vi "CreateIntegerArray.vi"(1 "Spacing":u16(ring) items=["Linear", "Logorithmic"], 2 "Pts":dbl, 3 "Max":dbl, 4 "Min":dbl) -> (0 "OutputArray":dbl[](array[numeric]))   [LabVIEW 2015]
uses:
  <vilib>/imath/engines/lvmath2/RunTimeSupport/NIMS_Complex To Real.vi
  <instcachedir>/0/NIMS_Complex To Real_01315F44AA8B4CE79FEF95AE999DC25E.lvgen/NIMS_Complex To Real_01315F44AA8B4CE79FEF95AE999DC25E_001.vi
  <vilib>/imath/engines/lvmath2/RunTimeEngine/BuiltInFunctions/logramp/NIMS_logramp.vi
  <vilib>/imath/engines/lvmath2/RunTimeEngine/ErrorHandling/NIMS_Create Error From Enums.vi
  <vilib>/imath/engines/lvmath2/RunTimeEngine/BuiltInFunctions/linramp/NIMS_linramp.vi
  <vilib>/imath/engines/lvmath2/RunTimeEngine/VariableToken/NIMS_VariableToken_CondDefined.vi
  <instcachedir>/0/NIMS_VariableToken_CondDefined_FE30D0A1BFB24F098D41DEBABFE96BE1.lvgen/NIMS_VariableToken_CondDefined_FE30D0A1BFB24F098D41DEBABFE96BE1_003.vi
  <vilib>/imathl/engines/lvmath/Functions/Error Handling/Create Error.vi
  <vilib>/imath/engines/lvmath2/RunTimeEngine/NodeEndStatement/NIMS_NodeEndStatement_Output.vi
  <instcachedir>/0/NIMS_NodeEndStatement_Output_53EC0D466D134D7ABD903AC30B43404B.lvgen/NIMS_NodeEndStatement_Output_53EC0D466D134D7ABD903AC30B43404B_005.vi
  <vilib>/imath/engines/lvmath2/RunTimeEngine/ErrorHandling/NIMS_Finalize Error.vi
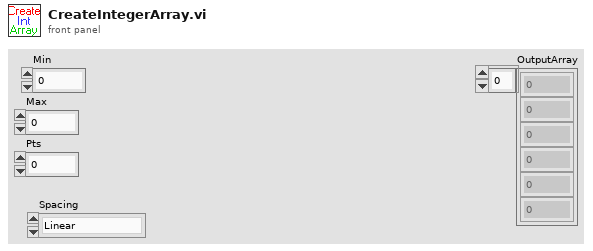
[diagram p1: front panel]
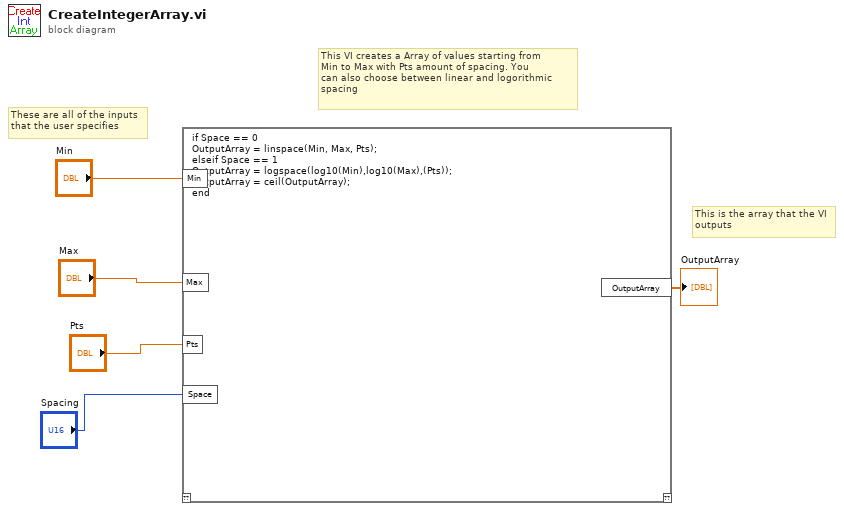
[diagram p0: block diagram]
diagram:
  # "This is the array that the VI\noutputs"
  # "These are all of the inputs\nthat the user specifies"
  # "This VI creates a Array of values starting from \nMin to Max with Pts amount of spacing. You \ncan also choose between linear and logorithmic \nspacing"
  n1 = mathscript code="if Space == 0\nOutputArray = linspace(Min, Max, Pts);\nelseif Space == 1\nOutputArray = logspace(log10(Min),log10(Max),(Pts));\nOutputArray = ceil(OutputArray);\nend"("Min"="Min", "Max"="Max", "Pts"="Pts", "Space"="Spacing") -> ("OutputArray"=→"OutputArray":dbl[])  [unwired: 1 in, 1 out]
